vi "Simple PID via Cryocon.vi"() -> ()   [LabVIEW 2016]
uses:
  <vilib>/addons/control/pid/pid.llb/PID (DBL).vi
  <vilib>/addons/control/pid/NI_PID_pid.lvlib
panel:
  out "resulting string":string
  out "VISA Resource Name Out":refnum<visa-resource-name>
  out "error out":errorcluster
  in  "error in (no error)":errorcluster
  in  "VISA Resource Name 2":refnum<visa-resource-name>
  in  "Stop":bool
  out "Process variable and Setpoint":cluster{"initial PV":dbl, "SP:":dbl}(graph)
  in  "PID gains":T1={"proportional gain (Kc)"=20.0, "integral time (Ti, min)"=0.008, "derivative time (Td, min)"=0.001} {"derivative time (Td, min)" format="%.3f"; "integral time (Ti, min)" format="%.3f"; "proportional gain (Kc)" format="%.3f"}
  out "PV:":dbl(slide)=60.754431603254424 scale=0.0..100.0
  in  "SP:":dbl(slide)=43.790849673202615 min=0.0 max=0.0 scale=0.0..100.0
  out "MV:":dbl(slide)=18.78965245852964 scale=-100.0..100.0
  out "Manipulated variable":dbl(graph)
  in  "VISA Resource Name":refnum<visa-resource-name>
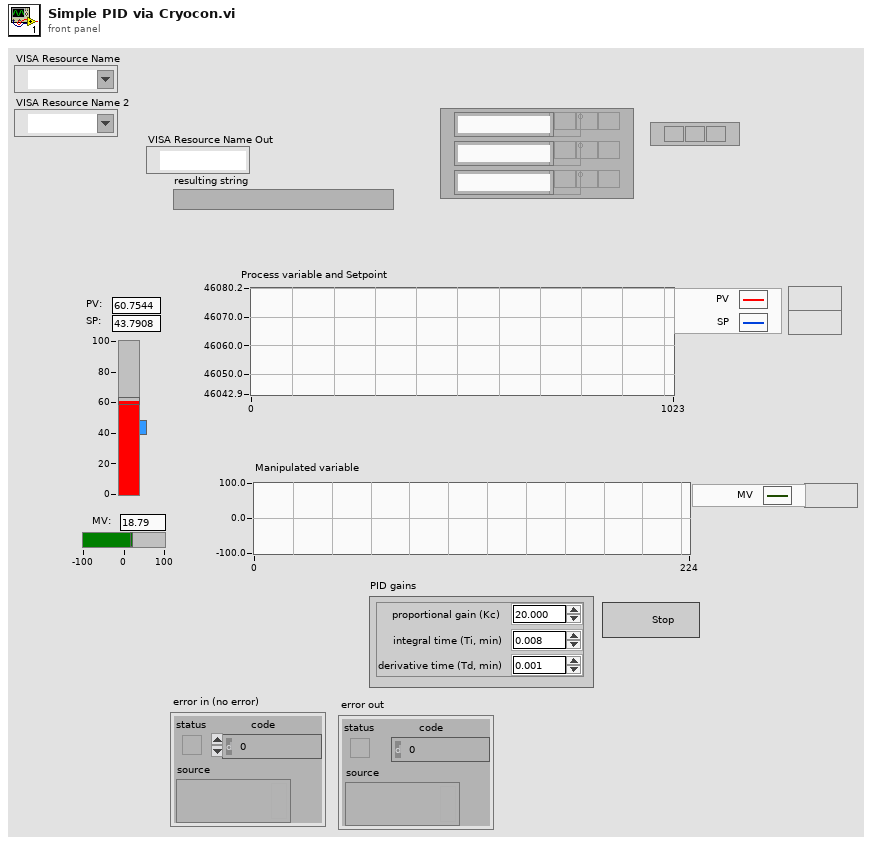
[diagram p1: front panel]
types:
  T1 = cluster{"proportional gain (Kc)":dbl, "integral time (Ti, min)":dbl, "derivative time (Td, min)":dbl}
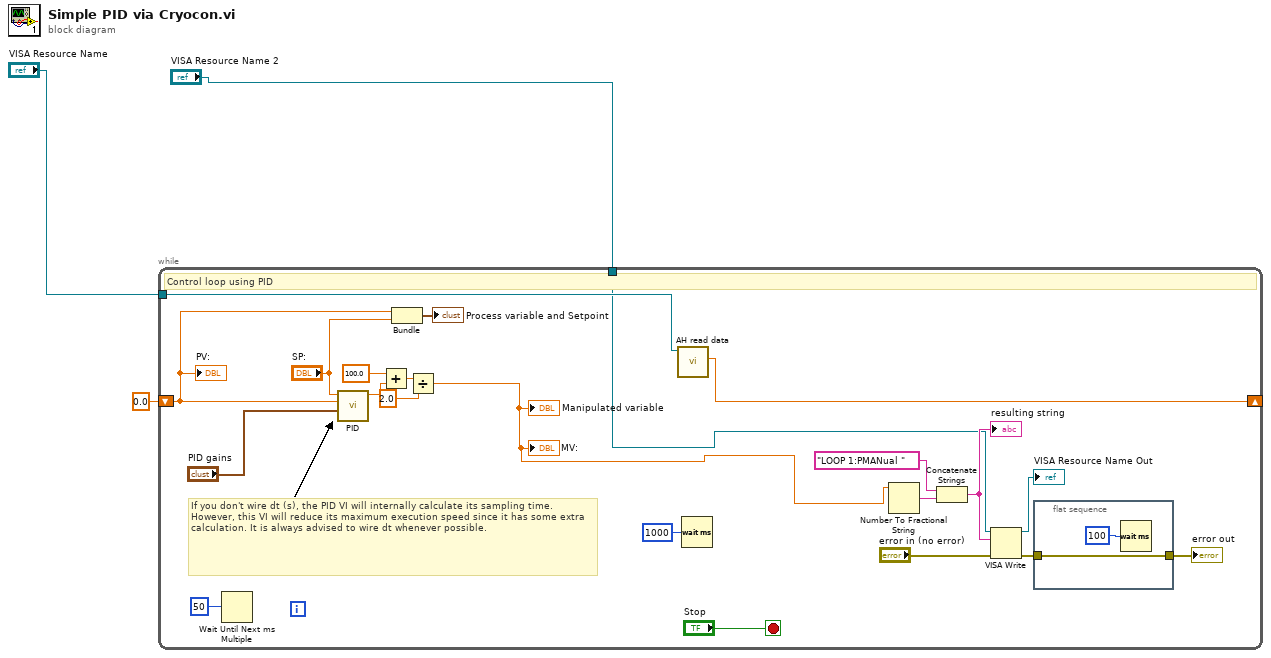
[diagram p0: block diagram]
diagram:
  n1 = while {
    shift-left: 0.0 ("Plant Output") -> [w23]
    shift-right: [w19] -> _
    tunnel: "VISA Resource Name" -> [w18]
    tunnel: "VISA Resource Name 2" -> [w5]
    stop <- "Stop" stop-if-true
    # "If you don't wire dt (s), the PID VI will internally calculate its sampling time. However, this VI will reduce its maximum execution speed since it has some extra calculation. It is always advised to wire dt whenever possible."
    # "Control loop using PID"
    n2 = Wait Until Next ms Multiple(millisecond multiple=u32 50 ("unsigned 32bit integer")) -> ()  [unwired: 1 out]
    n3 = call-poly <vilib>:"PID.vi"("PID gains"="PID gains", "process variable"=w23, "setpoint"="SP:") -> ("output"=w16:dbl)  [unwired: 7 in, 1 out]
    n4 = Add(x=100.0, y=w16) -> (x+y=w14:dbl)
    n5 = Bundle("Plant Output"=w23, "SP:"="SP:") -> (→"Process variable and Setpoint":cluster{"Plant Output":dbl, "SP:":dbl})  [unwired: 1 in]
    n6 = Divide(x=w14, y=2.0) -> (x/y=w4:dbl)
    "MV:" <- w4
    "Manipulated variable" <- w4
    n7 = call "AH read data.vi"("VISA Resource Name"=w18) -> ("Capacitance"=w19:dbl)  [unwired: 7 in, 3 out]
    n8 = Wait (ms)(milliseconds to wait=u32 1000) -> ()  [unwired: 1 out]
    n9 = Number To Fractional String(number=w4) -> (F-format string=w6:string)  [unwired: 3 in]
    n10 = Concatenate Strings("LOOP 1:PMANual " ("format string"), w6) -> (w8:string)
    "resulting string" <- w8
    n11 = VISA Write(VISA resource name=w5, write buffer=w8, error in (no error)="error in (no error)") -> (VISA resource name out=→"VISA Resource Name Out":refnum<visa-resource-name>, error out=w11:errorcluster)  [unwired: 1 out]
    n12 = flat-sequence {
      tunnel: w11 -> [w26]
      tunnel: [w26] -> w10
      frame #0 {
        n13 = Wait (ms)(milliseconds to wait=u32 100) -> ()  [unwired: 1 out]
      }
    }
    "PV:" <- w23
    "error out" <- w10
  }
